vi "Teardown.vi"(8 "Error In":errorcluster, 11 "Session":refnum<class "Session.lvclass">) -> (0 "Error Out":errorcluster)   [LabVIEW 2018, in "Tests.lvlib" / "Channel.lvlib"]
uses:
  Channel.lvlib
  src/Toolkit/API/Session/Session.lvclass
  src/Toolkit/API/SSH/SSH.lvclass
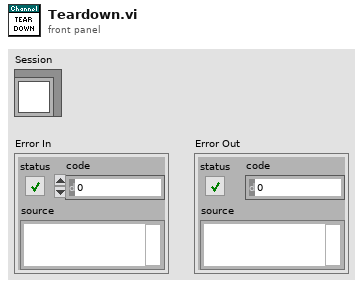
[diagram p1: front panel]
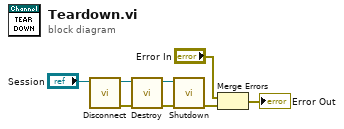
[diagram p0: block diagram]
diagram:
  n1 = call "Disconnect.vi"("Session In"="Session") -> ("Error Out"=w7:errorcluster, "Sesssion Out"=w6:refnum<class "Session.lvclass">)  [unwired: 9 in]
  n2 = call "Destroy.vi"("Error In"=w7, "Session"=w6) -> ("Error Out"=w4:errorcluster, "SSH"=w3:refnum<class "SSH.lvclass">)  [unwired: 8 in]
  n3 = call "Shutdown.vi"("Error In"=w4, "SSH"=w3) -> ("Error Out"=w5:errorcluster)  [unwired: 9 in]
  n4 = Merge Errors("Error In", w5) -> (→"Error Out":errorcluster)
